vi "get Front Panel control references.vi"(8 "error in (no error)":errorcluster, 10 "Signalling (Default: T)":bool=TRUE, 11 "Main VI":refnum<vi>) -> (0 "error out":errorcluster)   [LabVIEW 2012]
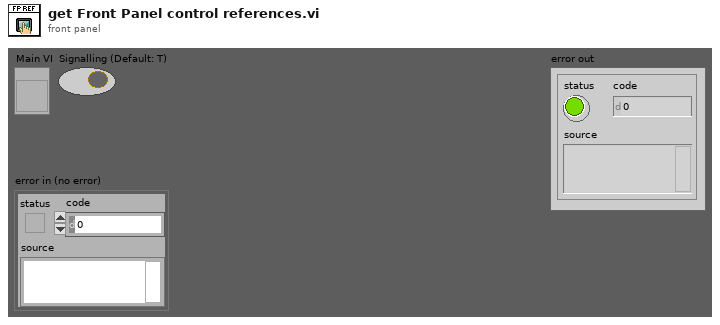
[diagram p1: front panel]
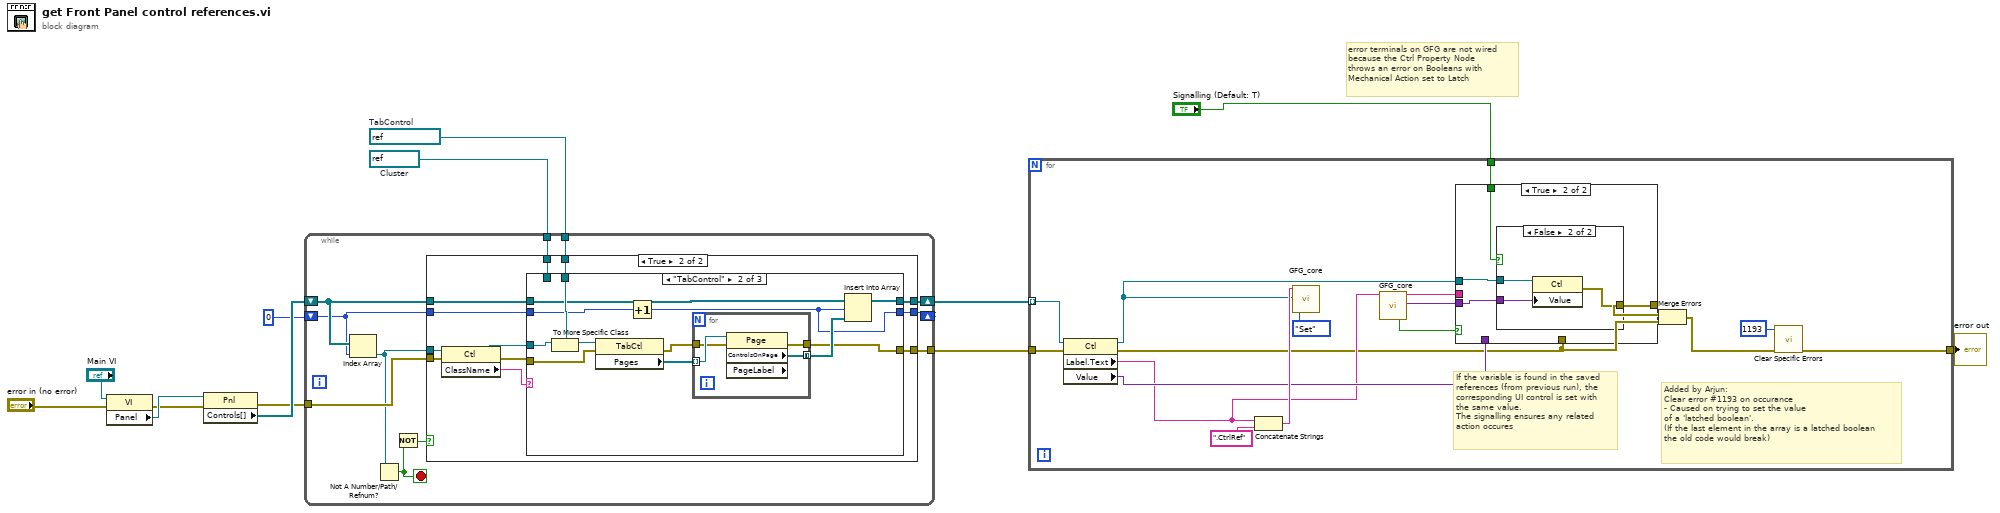
[diagram p0: block diagram]
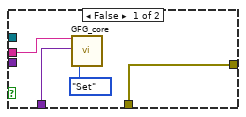
[diagram p2: hidden frame]
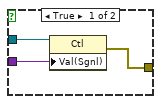
[diagram p3: hidden frame]
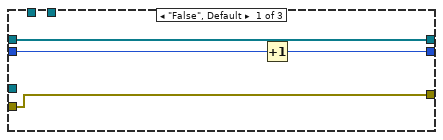
[diagram p5: hidden frame]
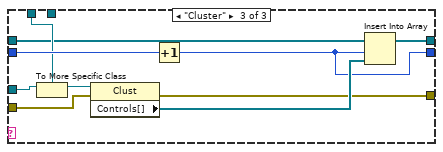
[diagram p6: hidden frame]
diagram:
  w4 = refnum<vi> refnum  # Cluster
  w11 = refnum<vi> refnum  # TabControl
  # "error terminals on GFG are not wired\nbecause the Ctrl Property Node\nthrows an error on Booleans with\nMechanical Action set to Latch"
  n1 = property class="VI"(reference="Main VI", error in="error in (no error)") -> (error out=w9:errorcluster, "Panel"=w13:refnum<vi>)  [unwired: 1 out]
  n2 = property class="Pnl"(reference=w13, error in=w9) -> (error out=w8:errorcluster, "Controls[]"=w12:refnum<vi>[])  [unwired: 1 out]
  n3 = while {
    shift-right: [w22] -> w7
    shift-left: w12 -> [w23]
    tunnel: w11 -> [w24]
    shift-right: [w20] -> _
    shift-left: 0 -> [w21]
    tunnel: w8 -> [w19]
    tunnel: w4 -> [w18]
    tunnel: [w15] -> w3
    stop <- w16 stop-if-true
    n4 = Index Array(array=w23, index=w21) -> (element=w14:refnum<vi>)
    n5 = Not A Number/Path/Refnum?(number/path/refnum=w14) -> (NaN/Path/Refnum?=w16:bool)
    n6 = Not(x=w16) -> (.not. x?=w17:bool)
    n7 = case shown="True" w17 {
      tunnel: w24 -> [_ w38]
      tunnel: w23 -> [w27 w37]
      tunnel: [w27 w36] -> w22
      tunnel: w21 -> [w26 w35]
      tunnel: [w26 w34] -> w20
      tunnel: w19 -> [w25 w33]
      tunnel: w18 -> [_ w31]
      tunnel: [w25 w30] -> w15
      tunnel: w14 -> [_ w29]
      frame False {
      }
      frame True {
        n8 = property class="Ctl"(reference=w29, error in=w33) -> (reference out=w39:refnum<vi>, error out=w32:errorcluster, "ClassName"=w28:string)
        n9 = case shown="\"TabControl\"" w28 {
          tunnel: w39 -> [_ w55 w69]
          tunnel: w38 -> [_ w54 _]
          tunnel: w37 -> [w43 w45 w61]
          tunnel: [w43 w50 w67] -> w36
          tunnel: w35 -> [w42 w46 w65]
          tunnel: [w41 w44 w60] -> w34
          tunnel: w32 -> [w40 w49 w66]
          tunnel: [w40 w47 w62] -> w30
          tunnel: w31 -> [_ _ w64]
          frame "False", Default {
            n10 = Increment(x=w42) -> (x+1=w41:i32)
          }
          frame "TabControl" {
            n11 = To More Specific Class(target class=w54, reference=w55) -> (specific class reference=w53:refnum<vi>)  [unwired: 1 in, 1 out]
            n12 = property class="TabCtl"(reference=w53, error in=w49) -> (error out=w48:errorcluster, "Pages"=w52:refnum<vi>[])  [unwired: 1 out]
            n13 = Increment(x=w46) -> (x+1=w44:i32)
            n14 = for {
              tunnel: w52 -> [w59] mode=indexing
              tunnel: [w58] -> w51 mode=concatenating
              tunnel: w48 -> [w57]
              tunnel: [w56] -> w47
              n15 = property class="Page" props=["ControlsOnPage", "PageLabel"](reference=w59, error in=w57) -> (error out=w56:errorcluster, "ControlsOnPage"=w58:refnum<vi>[])  [unwired: 2 out]
            }
            n16 = Insert Into Array(array=w45, index=w44, new element=w51) -> (w50:refnum<vi>[])
          }
          frame "Cluster" {
            n17 = To More Specific Class(target class=w64, reference=w69) -> (specific class reference=w68:refnum<vi>)  [unwired: 1 in, 1 out]
            n18 = property class="Clust"(reference=w68, error in=w66) -> (error out=w62:errorcluster, "Controls[]"=w63:refnum<vi>[])  [unwired: 1 out]
            n19 = Increment(x=w65) -> (x+1=w60:i32)
            n20 = Insert Into Array(array=w61, index=w60, new element=w63) -> (w67:refnum<vi>[])
          }
        }
      }
    }
  }
  n21 = for {
    tunnel: w7 -> [w83] mode=indexing
    tunnel: w3 -> [w85]
    tunnel: [w72] -> w2
    tunnel: "Signalling (Default: T)" -> [w70]
    # "If the variable is found in the saved references (from previous run), the  corresponding UI control is set with the same value.\nThe signalling ensures any related action occures"
    # "Added by Arjun:\nClear error #1193 on occurance\n- Caused on trying to set the value\nof a 'latched boolean'.\n(If the last element in the array is a latched boolean\nthe old code would break)"
    n22 = property class="Ctl"(reference=w83, error in=w85) -> (reference out=w76:refnum<vi>, error out=w74:errorcluster, "Label.Text"=w79:string, "Value"=w82:variant)
    n23 = Concatenate Strings(w79, ".CtrlRef" ("string")) -> (w84:string)
    n24 = call "GFG_core.vi"("Variable Name in"=w84, "Variant in"=w76, "Action"=enum16{"Init", "Set", "Get"}."Set") -> ()  [unwired: 10 in, 7 out]
    n25 = call "GFG_core.vi"("Variable Name in"=w79) -> ("Found/Replaced"=w80:bool, "Variable Name Out"=w78:string, "Variant Out"=w77:variant)  [unwired: 12 in, 4 out]
    n26 = case shown="True" w80 {
      tunnel: w82 -> [w90 _]
      tunnel: w78 -> [w88 _]
      tunnel: w77 -> [_ w93]
      tunnel: w76 -> [_ w94]
      tunnel: [w87 w92] -> w75
      tunnel: w74 -> [w87 _]
      tunnel: w70 -> [_ w91]
      frame False {
        n27 = call "GFG_core.vi"("Variable Name in"=w88, "Variant in"=w90, "Action"=enum16{"Init", "Set", "Get"}."Set") -> ()  [unwired: 10 in, 7 out]
      }
      frame True {
        n28 = case shown="False" w91 {
          tunnel: w94 -> [w97 w100]
          tunnel: w93 -> [w96 w99]
          tunnel: [w95 w98] -> w92
          frame True {
            n29 = property class="Ctl"(reference=w97, "Val(Sgnl)"=w96) -> (error out=w95:errorcluster)  [unwired: 1 in, 1 out]
          }
          frame False {
            n30 = property class="Ctl"(reference=w100, "Value"=w99) -> (error out=w98:errorcluster)  [unwired: 1 in, 1 out]
          }
        }
      }
    }
    n31 = Merge Errors(w75, w74) -> (w73:errorcluster)
    n32 = call "Clear Specific Errors.vi"("Error In"=w73, "Error number In"=1193) -> ("Error Out"=w72:errorcluster)  [unwired: 8 in, 1 out]
  }
  "error out" <- w2
